vi "temp chart scale adjust.vi"(0 "Control Parameters":T2={"Setpoint"=50.0, "Control bandwidth"=4.0, "Settle bandwidth"=1.0} {"Settle bandwidth" format="%.2f"; "Control bandwidth" format="%.2f"; "Setpoint" format="%.2f"}, 7 "Scale Control In":T1, 9 "Temperature History":refnum<vi>) -> (8 "Scale Control Out":T1, 10 "Temperature History out":refnum<vi>)   [LabVIEW 2014]
doc: "This subvi adjusts the scales on the temperature chart.\n\nPaul K Dixon\nPhysics 350\nCSUSB Physics"
panel:
  # "scale adjust"
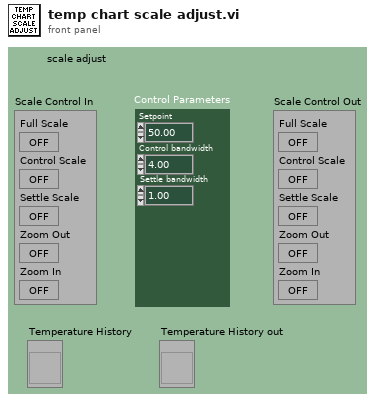
[diagram p1: front panel]
types:
  T1 = cluster{"Full Scale":bool, "Control Scale":bool, "Settle Scale":bool, "Zoom Out":bool, "Zoom In":bool}
  T2 = cluster{"Setpoint":dbl, "Control bandwidth":dbl, "Settle bandwidth":dbl}
  T3 = cluster{"temp out":dbl, dbl, dbl, dbl, dbl, dbl, dbl}[]
  T4 = cluster{"temp out":dbl, dbl, dbl, dbl, dbl, dbl, dbl}
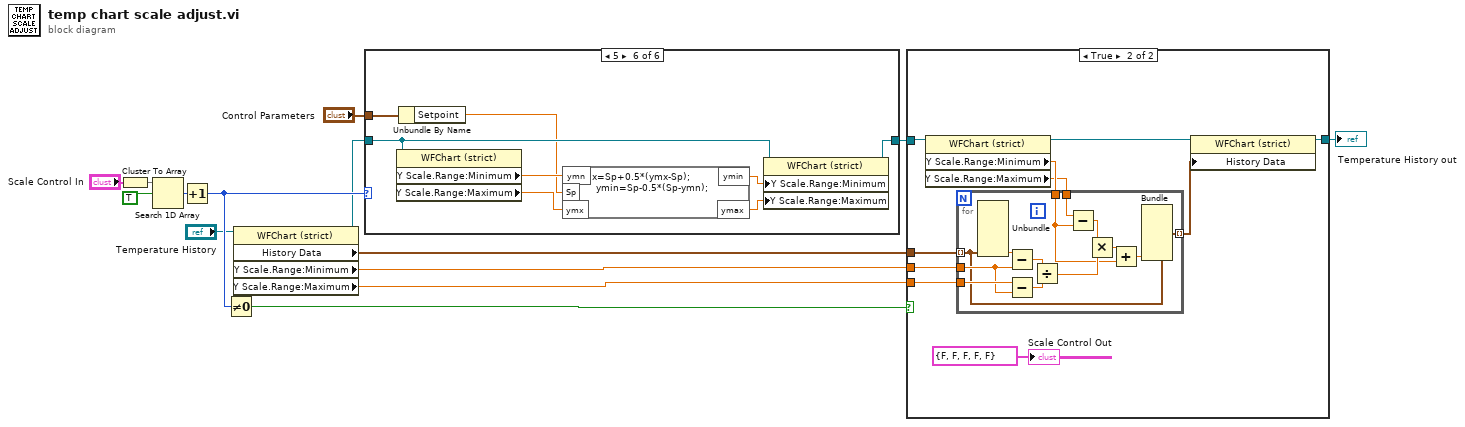
[diagram p0: block diagram]
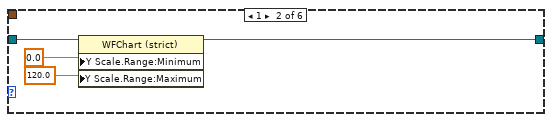
[diagram p4: hidden frame]
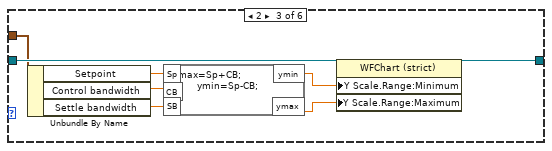
[diagram p5: hidden frame]
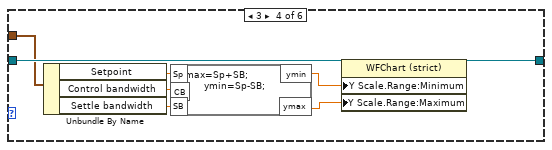
[diagram p6: hidden frame]
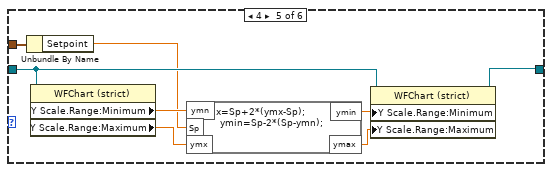
[diagram p7: hidden frame]
diagram:
  n1 = Cluster To Array(cluster="Scale Control In") -> (array=w12:bool[])
  n2 = Search 1D Array(1D array=w12, element=TRUE) -> (index of element=w14:i32)  [unwired: 1 out]
  n3 = Increment(x=w14) -> (x+1=w10:i32)
  n4 = Not Equal To 0?(x=w10) -> (x != 0?=w7:bool)
  n5 = property on="Property Node" class="WFChart (strict)"(reference="Temperature History") -> (reference out=w9:refnum<vi>, "History Data"=w4:T3, "Y Scale.Range:Minimum"=w6:dbl, "Y Scale.Range:Maximum"=w5:dbl)  [unwired: 1 in, 1 out]
  n6 = case shown="5" w10 {
    tunnel: "Control Parameters" -> [_ _ w23 w31 w37 w45]
    tunnel: w9 -> [w15 w17 w25 w33 w39 w46]
    tunnel: [w15 w16 w24 w32 w38 w47] -> w8
    frame 0, Default {
    }
    frame 1 {
      n7 = property on="Property Node" class="WFChart (strict)"(reference=w17, "Y Scale.Range:Minimum"=0.0, "Y Scale.Range:Maximum"=120.0) -> (reference out=w16:refnum<vi>)  [unwired: 1 in, 1 out]
    }
    frame 2 {
      n8 = Unbundle By Name(w23) -> ("Setpoint"=w22:dbl, "Control bandwidth"=w21:dbl, "Settle bandwidth"=w20:dbl)
      n9 = formula code="ymax=Sp+CB;\n        ymin=Sp-CB;"("Sp"=w22, "CB"=w21, "SB"=w20) -> ("ymax"=w26:dbl, "ymin"=w27:dbl)
      n10 = property on="Property Node" class="WFChart (strict)"(reference=w25, "Y Scale.Range:Minimum"=w27, "Y Scale.Range:Maximum"=w26) -> (reference out=w24:refnum<vi>)  [unwired: 1 in, 1 out]
    }
    frame 3 {
      n11 = Unbundle By Name(w31) -> ("Setpoint"=w30:dbl, "Control bandwidth"=w29:dbl, "Settle bandwidth"=w28:dbl)
      n12 = formula code="ymax=Sp+SB;\n        ymin=Sp-SB;"("Sp"=w30, "CB"=w29, "SB"=w28) -> ("ymax"=w34:dbl, "ymin"=w35:dbl)
      n13 = property on="Property Node" class="WFChart (strict)"(reference=w33, "Y Scale.Range:Minimum"=w35, "Y Scale.Range:Maximum"=w34) -> (reference out=w32:refnum<vi>)  [unwired: 1 in, 1 out]
    }
    frame 4 {
      n14 = Unbundle By Name(w37) -> ("Setpoint"=w36:dbl)
      n15 = property on="Property Node" class="WFChart (strict)"(reference=w39) -> ("Y Scale.Range:Minimum"=w41:dbl, "Y Scale.Range:Maximum"=w40:dbl)  [unwired: 1 in, 2 out]
      n16 = formula code="ymax=Sp+2*(ymx-Sp);\n        ymin=Sp-2*(Sp-ymn);"("ymn"=w41, "Sp"=w36, "ymx"=w40) -> ("ymax"=w42:dbl, "ymin"=w43:dbl)
      n17 = property on="Property Node" class="WFChart (strict)"(reference=w39, "Y Scale.Range:Minimum"=w43, "Y Scale.Range:Maximum"=w42) -> (reference out=w38:refnum<vi>)  [unwired: 1 in, 1 out]
    }
    frame 5 {
      n18 = property on="Property Node" class="WFChart (strict)"(reference=w46) -> ("Y Scale.Range:Minimum"=w49:dbl, "Y Scale.Range:Maximum"=w48:dbl)  [unwired: 1 in, 2 out]
      n19 = Unbundle By Name(w45) -> ("Setpoint"=w44:dbl)
      n20 = formula code="ymax=Sp+0.5*(ymx-Sp);\n        ymin=Sp-0.5*(Sp-ymn);"("ymn"=w49, "Sp"=w44, "ymx"=w48) -> ("ymax"=w50:dbl, "ymin"=w51:dbl)
      n21 = property on="Property Node" class="WFChart (strict)"(reference=w46, "Y Scale.Range:Minimum"=w51, "Y Scale.Range:Maximum"=w50) -> (reference out=w47:refnum<vi>)  [unwired: 1 in, 1 out]
    }
  }
  n22 = case shown="True" w7 {
    tunnel: w8 -> [w52 w62]
    tunnel: w4 -> [_ w60]
    tunnel: w6 -> [_ w59]
    tunnel: w5 -> [_ w58]
    tunnel: [w52 w54] -> w2
    frame False {
    }
    frame True {
      n23 = property on="Property Node" class="WFChart (strict)"(reference=w62) -> (reference out=w61:refnum<vi>, "Y Scale.Range:Minimum"=w57:dbl, "Y Scale.Range:Maximum"=w56:dbl)  [unwired: 1 in, 1 out]
      n24 = for {
        tunnel: w60 -> [w65] mode=indexing
        tunnel: w59 -> [w73]
        tunnel: w58 -> [w74]
        tunnel: w57 -> [w67]
        tunnel: w56 -> [w70]
        tunnel: [w63] -> w55 mode=indexing
        n25 = Unbundle(w65) -> (w75:dbl)  [unwired: 6 out]
        n26 = Subtract(x=w75, y=w73) -> (x-y=w72:dbl)
        n27 = Subtract(x=w74, y=w73) -> (x-y=w71:dbl)
        n28 = Divide(x=w72, y=w71) -> (x/y=w68:dbl)
        n29 = Subtract(x=w70, y=w67) -> (x-y=w69:dbl)
        n30 = Multiply(x=w69, y=w68) -> (x*y=w66:dbl)
        n31 = Add(x=w66, y=w67) -> (x+y=w64:dbl)
        n32 = Bundle(cluster=w65, w64) -> (w63:T4)  [unwired: 6 out]
      }
      n33 = property on="Property Node" class="WFChart (strict)"(reference=w61, "History Data"=w55) -> (reference out=w54:refnum<vi>)  [unwired: 1 in, 1 out]
      "Scale Control Out" <- T1 {"Full Scale"=FALSE, "Control Scale"=FALSE, "Settle Scale"=FALSE, "Zoom Out"=FALSE, "Zoom In"=FALSE} ("Scale Control Out")
    }
  }
  "Temperature History out" <- w2
